vi "Error Queue Next.vi"(8 "error in (no error)":errorcluster, 10 "Node In":string, 11 "VISA resource name":refnum<visa-resource-name>) -> (0 "error out":errorcluster, 1 "Next Error":string, 2 "Node  Out":string, 3 "VISA resource name out":refnum<visa-resource-name>, 4 "Command String":string)   [LabVIEW 2012, in "Keithley 2600 Series.lvlib"]
doc: "Reads an entry from the error/event queue.\n\n<b>Remarks:</b>\nThis VI performs the same operation as Error Query however, rather than returning errors via error out it returns the exact output of the instrument.\n\n<b>Functions and Attributes Used</b>\nerrorqueue.next()"
uses:
  Keithley 2600 Series.lvlib
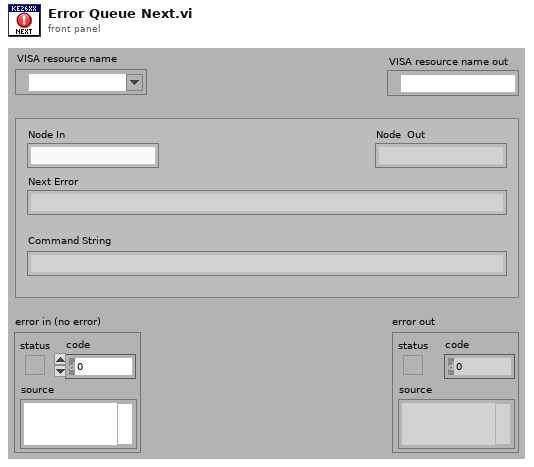
[diagram p1: front panel]
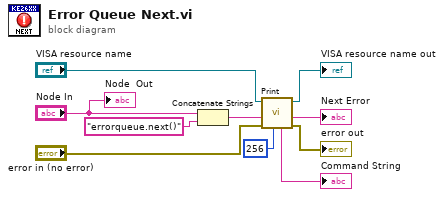
[diagram p0: block diagram]
diagram:
  n1 = Concatenate Strings("Node In", "errorqueue.next()" ("command")) -> (w8:string)
  n2 = call "Print.vi"("Byte Count (1024)"=u32 256, "error in (no error)"="error in (no error)", "Input"=w8, "VISA resource name"="VISA resource name") -> ("error out"=→"error out":errorcluster, "Output"=→"Next Error":string, "VISA resource name out"=→"VISA resource name out":refnum<visa-resource-name>, "Command String"=→"Command String":string)  [unwired: 1 in, 3 out]
  "Node  Out" <- "Node In"
